vi "Reset Test Status.vi"(8 "error in (no error)":errorcluster, 11 "Model in":refnum<class "Model.lvclass">) -> (0 "error out":errorcluster, 3 "Model out":refnum<class "Model.lvclass">)   [LabVIEW 2016, in "Model.lvclass"]
uses:
  Model.lvclass
  Typedefs/AllTestStatus.ctl
  Typedefs/TestStatus.ctl
  Model.lvclass/Model.ctl
  Typedefs/FAMT Typedefs.lvlib
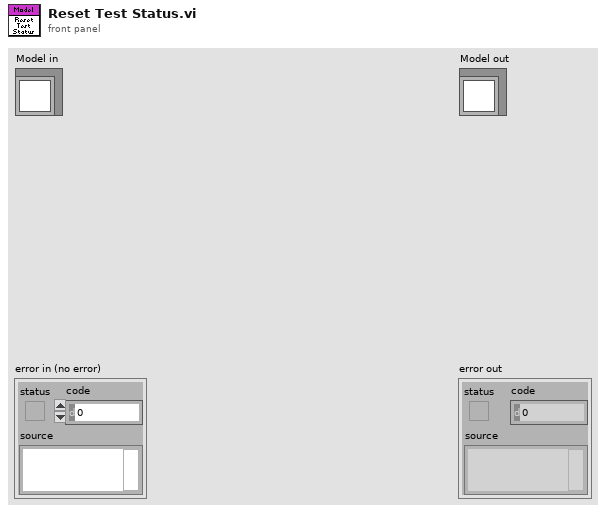
[diagram p1: front panel]
types:
  T1 = typedef "FAMT Typedefs.lvlib/AllTestStatus.ctl" = cluster{"Differential Pressure Release Valve Test":T2, "Force Accuracy Test":T2, "Full Force Test":T2, "Operational Force Test":T2, "Sentran Accuracy Test":T2, "Slewing Test":T2, "Tracking Test":T2, "Zero Force Test":T2}
  T2 = typedef "FAMT Typedefs.lvlib/TestStatus.ctl" = enum16{"Not Run", "Running", "Passed", "Failed"}
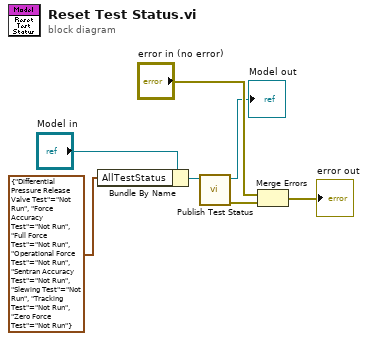
[diagram p0: block diagram]
diagram:
  n1 = Bundle By Name(cluster="Model in", "AllTestStatus"=T1 {"Differential Pressure Release Valve Test"=enum."Not Run", "Force Accuracy Test"=enum."Not Run", "Full Force Test"=enum."Not Run", "Operational Force Test"=enum."Not Run", "Sentran Accuracy Test"=enum."Not Run", "Slewing Test"=enum."Not Run", "Tracking Test"=enum."Not Run", "Zero Force Test"=enum."Not Run"}) -> (w3:refnum<class "Model.lvclass">)
  n2 = call "Publish Test Status.vi"("Model in"=w3) -> ("error out"=w1:errorcluster, "Model out"=→"Model out":refnum<class "Model.lvclass">)  [unwired: 9 in]
  n3 = Merge Errors("error in (no error)", w1) -> (→"error out":errorcluster)
